vi "TestVI.vi"(11 "Numeric":i32=3) -> (2 "String":string="Done", 3 "Boolean":bool)   [LabVIEW 2024]
panel:
  in  "String 2":string
  in  "OK Button":bool
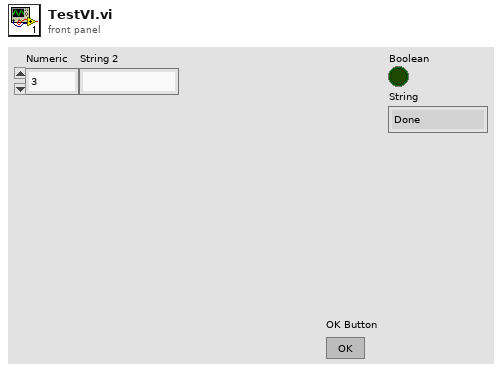
[diagram p1: front panel]
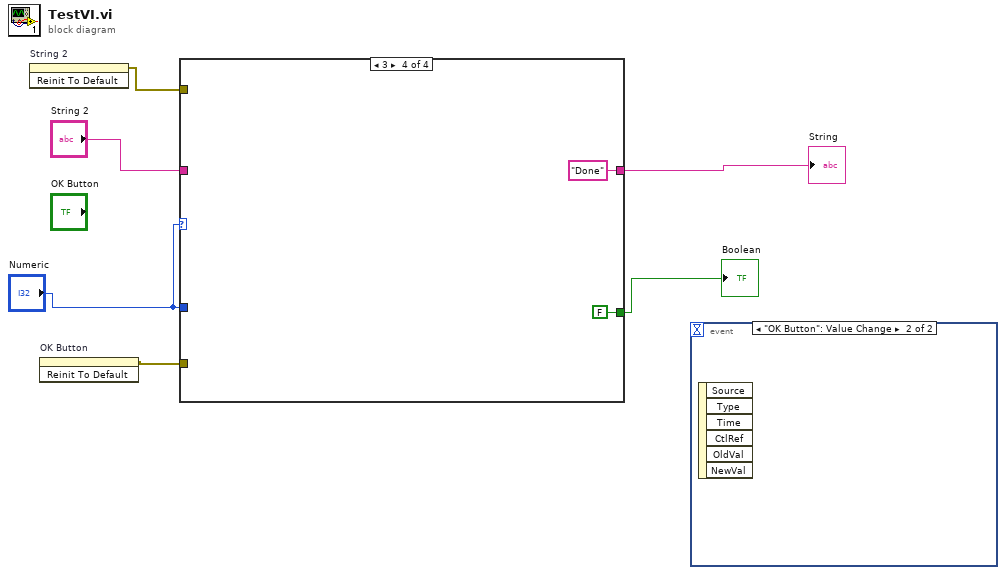
[diagram p0: block diagram]
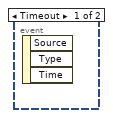
[diagram p2: hidden frame]
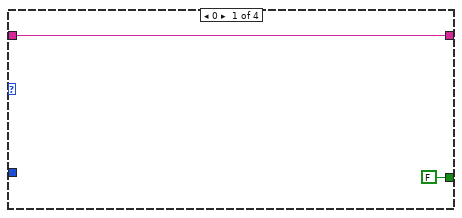
[diagram p3: hidden frame]
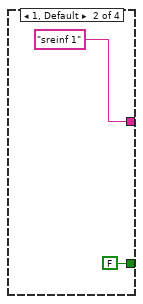
[diagram p4: hidden frame]
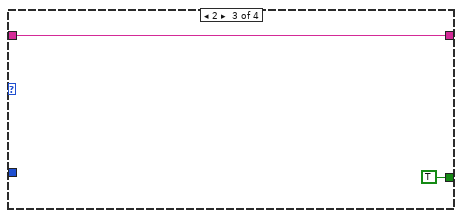
[diagram p5: hidden frame]
diagram:
  n1 = invoke on="String 2" class="Str" method="Reinit To Default"() -> (error out=w2:errorcluster)  [unwired: 3 in, 2 out]
  n2 = invoke on="OK Button" class="Bool" method="Reinit To Default"() -> (error out=w1:errorcluster)  [unwired: 3 in, 2 out]
  n3 = case shown="3" "Numeric" {
    tunnel: "Numeric" -> [_ _ _ _]
    tunnel: [FALSE FALSE TRUE FALSE] -> w4
    tunnel: [w7 "sreinf 1" w11 "Done" ("String 2")] -> w6
    tunnel: "String 2" -> [w7 _ w11 _]
    tunnel: w2 -> [_ _ _ _]
    tunnel: w1 -> [_ _ _ _]
    frame 0 {
    }
    frame 1, Default {
    }
    frame 2 {
    }
    frame 3 {
    }
  }
  "Boolean" <- w4
  "String" <- w6
  n4 = event shown="[1] \"OK Button\": Value Change" {
    selector: _ -> [_ _]
    dyn-events: _ -> [_ _]
    timeout: _ -> [_ _]
    event Timeout {
      n5 = event-data() -> ()  [unwired: 1 in, 3 out]
    }
    event "OK Button": Value Change {
      n6 = event-data() -> ()  [unwired: 1 in, 6 out]
    }
  }
